vi "Read CurrentPCFG.vi"(8 "Error In":errorcluster, 11 "INI Refnum":T1) -> (0 "Error Out":errorcluster, 1 "Config File Exists?":bool, 2 "Path Out":path)   [LabVIEW 2014, in "Standard Editor.lvlib"]
doc: "Read CurrentPCFG token from INI file and report whether the file exists"
uses:
  Standard Editor.lvlib
  <vilib>/Utility/config.llb/Config Data RefNum.ctl
  <vilib>/Utility/config.llb/Read Key (Path).vi
  <vilib>/Utility/config.llb/NI_LVConfig.lvlib
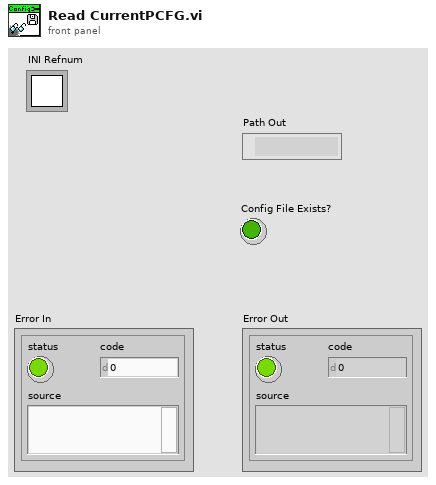
[diagram p1: front panel]
types:
  T1 = typedef "NI_LVConfig.lvlib/Config Data RefNum.ctl" = refnum<k1>
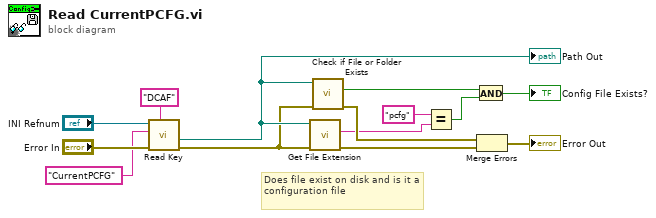
[diagram p0: block diagram]
diagram:
  # "Does file exist on disk and is it a configuration file"
  n1 = call-poly <vilib>:"Read Key.vi"("section"="DCAF", "error in (no error)"="Error In", "key"="CurrentPCFG", "refnum"="INI Refnum") -> ("error out"=w11:errorcluster, "value"=w12:path)  [unwired: 4 in, 2 out]
  "Path Out" <- w12
  n2 = call <vilib>:"Get File Extension.vi"("error in (no error)"=w11, "file"=w12) -> ("error out"=w10:errorcluster, "lowercase file extension"=w6:string)  [unwired: 6 in, 2 out]
  n3 = call <vilib>:"Check if File or Folder Exists.vi"("error in (no error)"=w11, "path"=w12) -> ("error out"=w9:errorcluster, "file or folder exists?"=w7:bool)  [unwired: 7 in, 1 out]
  n4 = Equal?(x="pcfg", y=w6) -> (x = y?=w4:bool)
  n5 = And(x=w7, y=w4) -> (x .and. y?=→"Config File Exists?":bool)
  n6 = Merge Errors(w9, w10) -> (→"Error Out":errorcluster)
